vi "convert data.vi"(7 "Data Type":T1, 11 "trimmed string":string) -> (3 "Data":T2)   [LabVIEW 2017]
uses:
  Type defs/data type.ctl
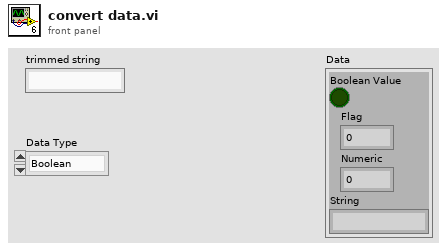
[diagram p1: front panel]
types:
  T1 = typedef "data type.ctl" = enum16{"Boolean", "Flag", "Numeric", "String", "Array"}
  T2 = cluster{"Boolean Value":bool, "Flag":i32, "Numeric":dbl, "String":string}
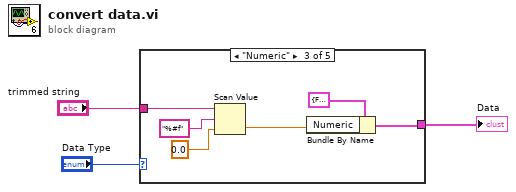
[diagram p0: block diagram]
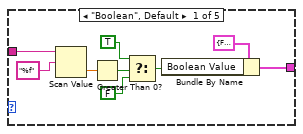
[diagram p2: hidden frame]
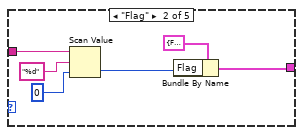
[diagram p3: hidden frame]
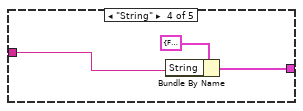
[diagram p4: hidden frame]
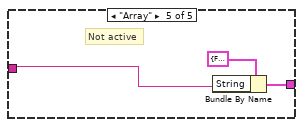
[diagram p5: hidden frame]
diagram:
  n1 = case shown="\"Numeric\"" "Data Type" {
    tunnel: "trimmed string" -> [w11 w17 w20 w26 w28]
    tunnel: [w4 w13 w19 w25 w29] -> w2
    frame "Boolean", Default {
      n2 = Scan Value(string=w11, format string="%f") -> (value=w10:dbl)  [unwired: 1 in, 1 out]
      n3 = Greater Than 0?(x=w10) -> (x > 0?=w9:bool)
      n4 = Select(t=TRUE, s=w9, f=FALSE) -> (s? t:f=w6:bool)
      n5 = Bundle By Name(cluster=T2 {"Boolean Value"=FALSE, "Flag"=0, "Numeric"=0.0, "String"=""} ("Data"), "Boolean Value"=w6) -> (w4:T2)
    }
    frame "Flag" {
      n6 = Scan Value(string=w17, format string="%d", default (0 dbl)=0) -> (value=w14:i32)  [unwired: 1 out]
      n7 = Bundle By Name(cluster=T2 {"Boolean Value"=FALSE, "Flag"=0, "Numeric"=0.0, "String"=""} ("Data"), "Flag"=w14) -> (w13:T2)
    }
    frame "Numeric" {
      n8 = Scan Value(string=w20, format string="%#f", default (0 dbl)=0.0) -> (value=w21:dbl)  [unwired: 1 out]
      n9 = Bundle By Name(cluster=T2 {"Boolean Value"=FALSE, "Flag"=0, "Numeric"=0.0, "String"=""} ("Data"), "Numeric"=w21) -> (w19:T2)
    }
    frame "String" {
      n10 = Bundle By Name(cluster=T2 {"Boolean Value"=FALSE, "Flag"=0, "Numeric"=0.0, "String"=""} ("Data"), "String"=w26) -> (w25:T2)
    }
    frame "Array" {
      # "Not active"
      n11 = Bundle By Name(cluster=T2 {"Boolean Value"=FALSE, "Flag"=0, "Numeric"=0.0, "String"=""} ("Data"), "String"=w28) -> (w29:T2)
    }
  }
  "Data" <- w2
